vi "main_control_combo_F.vi"(6 "read":bool) -> (9 "chiller actual temperature (C)":string, 10 "bytes read":u32)   [LabVIEW 2019]
doc: "The Basic Serial Read and Write example performs a Serial Port Read, a Serial Port Write, or a combination of these actions. The user selects the actions (read or write) on the front panel. If both are selected, the VI will write the data first, read data, and then close the VISA session that is opened to the port. This VI will wait until the specified number of bytes is received at the port. Only the number of bytes specified will be read.\n\nINSTRUCTIONS:\n1) Select the serial resource and configuration parameters (baud rate, data bits, parity, stop bits, flow control).\n2) Select the operations to be performed. \n3) Connect the serial port to your device. If no device is available, perform a loopback test by doing one of the following. Short pins 2 and 3 on a RS-232 cable or short pin 4 to pin 8 and pin 5 to pin 9 on a RS-485/422 cable. \n4) Run the VI to see the data read. (The \"read string\" will match the \"string to write\" if a loopback test was performed.)\n\nNote: The parameters set for the serial port must match the parameters of the connected instrument or device. In this example, the bytes to read parameter specifies the number of bytes that the serial port reads. If there were more bytes at the port than the number specified in bytes to read, those bytes would not be read. Also, if you specify to read more bytes than the number of bytes actually read, you might receive a timeout error message.\n\nOn the block diagram, the Configure Serial Port VI sets the configuration parameters. The front panel displays the controls used to configure the basic parameters, such as baud rate, data bits, and parity. Constants configure the other parameters the user probably does not need set. After the VISA Configure Serial Port VI opens the VISA session and configures the port, the VI passes the VISA resource name to other VIs that perform operations on that VISA resource. The VISA Write function sends a command to the serial device and the VISA Read function returns data based on the command. The VISA Close function then closes the reference to the serial device. It is important to close the reference; otherwise communication through with that port through protocols other than VISA might not be possible."
uses:
  <vilib>/Instr/_visa.llb/VISA Configure Serial Port (Instr).vi
  <vilib>/Utility/file.llb/Read Delimited Spreadsheet (string).vi
  Keithley/Keithley 24XX/Public/Data/Read (Single Point).vi
  Keithley/Keithley 24XX/Keithley 24XX.lvlib
  <resource>/objmgr/ni.var.rc
panel:
  out "DAQ readout from Linux Box":string
  in  "Output voltage (V)":dbl
  in  "Compliance (A)":dbl=1e-05
  in  "enable manual set":bool
  in  "Reset (default: false)":bool
  out "Finished times":i32
  in  "run single command":bool
  in  "command row":string[](array[string])
  in  "read 4":bool
  in  "read rotronic log manually":bool
  in  "Times to run script":i32=1 caption="times to run script"
  out "COMBO COMMAND":string
  out "manual control":bool
  out "delta actual voltage (V)":string
  in  "delay before read (ms) 4":u32=500
  in  "Combo Box 4":string(combo)
  in  "voltage delta":dbl
  out "delta command":string
  in  "write 4":bool
  in  "stop reading script":bool
  out "dewpoint":string
  out "temperature":string
  out "humidity":string
  out "Voltage (V)":sgl
  out "Current (A)":sgl
  out "Resistance (Om)":sgl
  out "Current (micro amps)":sgl
  out "Command Log and Output":string
  out "all rows":string[][](array[string])
  out "current command":string[](array[string])
  in  "CSV script path":path
  in  "Read Script":bool
  out "relay TTi":errorcluster
  out "bytes read 3":u32
  out "inverter actual voltage":string
  in  "read 3":bool
  in  "delay before read (ms) 3":u32=500
  in  "Combo Box of inverter":string(combo)="VO?\n"
  in  "voltage or current 2":dbl
  out "string from combo 3":string
  in  "write 3":bool
  out "LV TTi":errorcluster
  out "bytes read 2":u32
  out "LVPS actual voltage":string
  in  "read 2":bool
  in  "delay before read (ms) 2":u32=500
  in  "Combo Box of TTi LVPS":string(combo)="VO?\n"
  in  "voltage or current":dbl
  in  "write 2":bool
  in  "write":bool
  out "string from combo":string
  in  "Set Temperature":dbl
  in  "Combo Box of chiller":string(combo)
  out "Chiller":errorcluster
  out "N2 temperature > dew point + 5C":bool
  in  "File Path of rotonic datalog":path
  out "time humidity temporature dewpoint":string[](array[string])
  in  "Quit":bool
  in  "delay before read (ms)":u32=500
  # "Please click \"Reset\" to \"True\" ONLY AFTER Keithley is power cycled\n(BEFORE launching the VI)"
  # "Kiethley Powersupply"
  # "µA"
  # "Delta powersupply Interface"
  # "Medical Chiller\nCOM 6 is default"
  # "TTi LV powersupply\nCOM 5 is default"
  # "TTi LV powersupply for the relay polarity control\nCOM 4 is default"
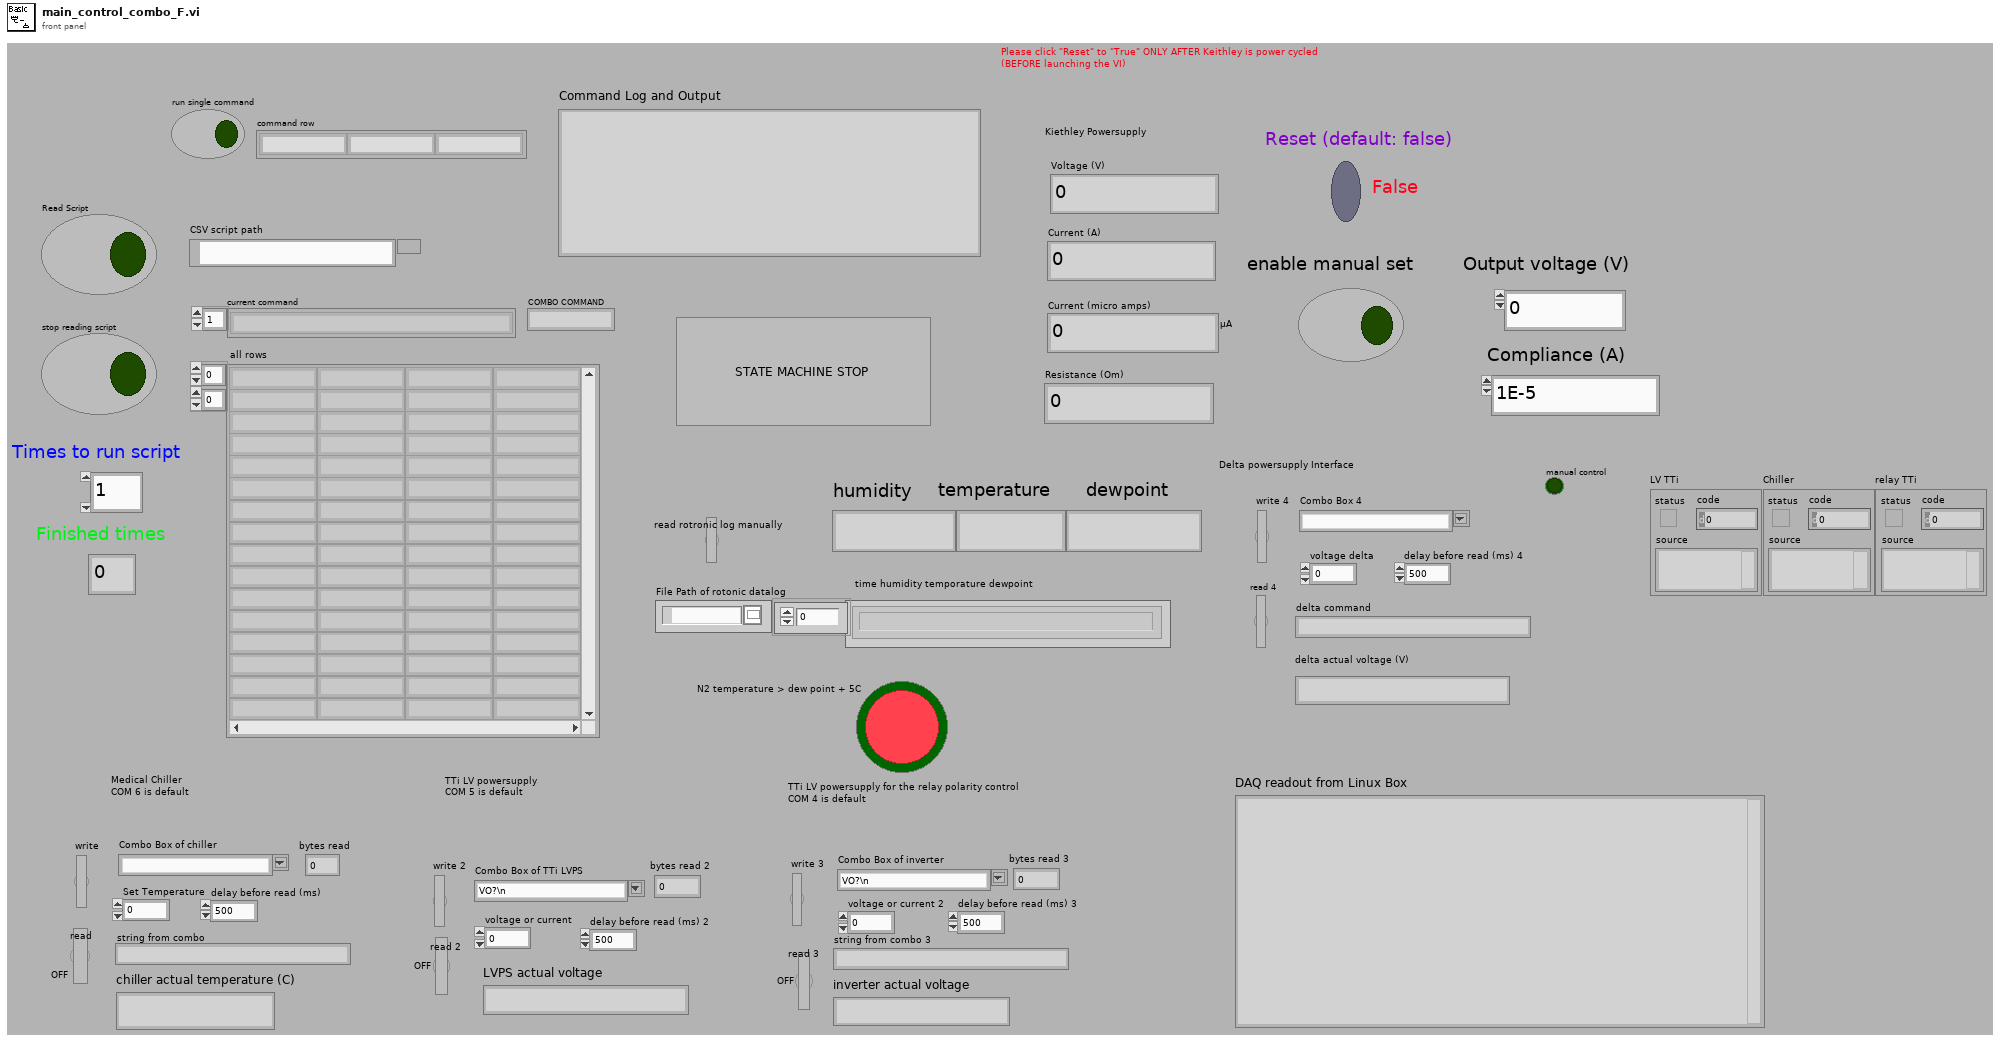
[diagram p1: front panel]
types:
  T1 = cluster{"Baud Rate":u32, "Parity":u16, "Data Bits":u16, "Stop Bits":u16, "Flow Control":u16}
  T2 = enum16{"open", "replace", "create", "open or create", "replace or create", "replace or create with confirmation"}
  T3 = typedef "Semaphore RefNum" = refnum<k1>
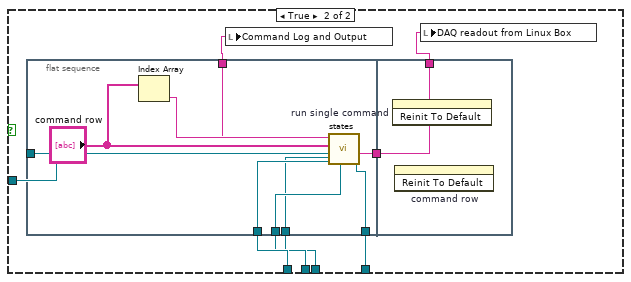
[diagram p3: hidden frame]
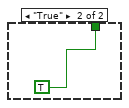
[diagram p4: hidden frame]
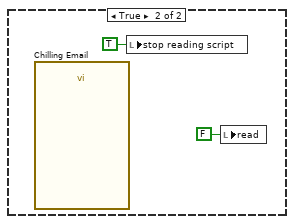
[diagram p6: hidden frame]
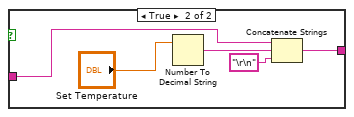
[diagram p7: hidden frame]
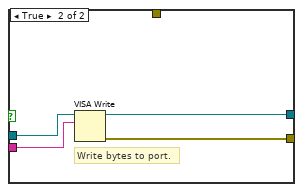
[diagram p8: hidden frame]
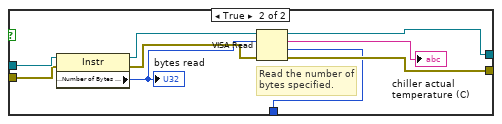
[diagram p9: hidden frame]
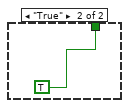
[diagram p10: hidden frame]
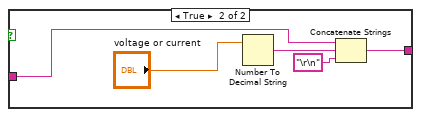
[diagram p12: hidden frame]
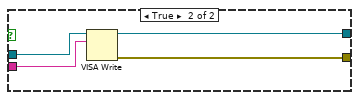
[diagram p13: hidden frame]
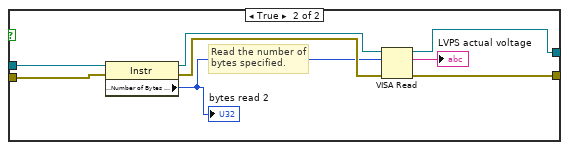
[diagram p14: hidden frame]
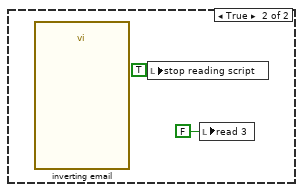
[diagram p16: hidden frame]
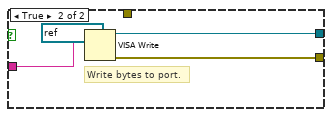
[diagram p18: hidden frame]
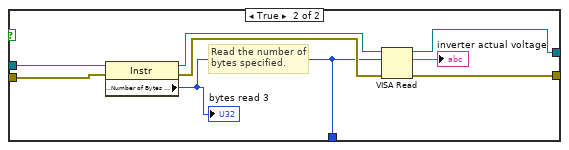
[diagram p19: hidden frame]
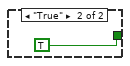
[diagram p20: hidden frame]
diagram:
  # "First save permanent values in non-volatile memory via NI - Max and the *SAV after setting it via SO:VO:MA 52 and SO:CU:MA 30    !"
  n1 = flat-sequence {
    tunnel: [w26] -> w16
    tunnel: [w40] -> w15
    tunnel: [w28] -> w14
    tunnel: [w34] -> w13
    tunnel: [w33] -> w12
    tunnel: [w29] -> w11
    tunnel: [w29] -> w10
    tunnel: [w25] -> w9
    tunnel: [w24] -> w8
    tunnel: [w23] -> w7
    tunnel: [w25] -> w6
    tunnel: [w24] -> w5
    tunnel: [w23] -> w4
    tunnel: [w20] -> w3
    tunnel: [w20] -> w2
    tunnel: [w20] -> w1
    tunnel: [w62] -> w19
    tunnel: [w61] -> w17
    tunnel: w16 -> [w60]
    tunnel: w15 -> [_]
    tunnel: w14 -> [w59]
    tunnel: w13 -> [w57]
    tunnel: w12 -> [w58]
    tunnel: w11 -> [w52]
    tunnel: w10 -> [w56]
    tunnel: w9 -> [w51]
    tunnel: w8 -> [w50]
    tunnel: w7 -> [w49]
    tunnel: w6 -> [w55]
    tunnel: w5 -> [w54]
    tunnel: w4 -> [w53]
    tunnel: w3 -> [w48]
    tunnel: w2 -> [w47]
    tunnel: w1 -> [w46]
    tunnel: w19 -> [w594]
    tunnel: w17 -> [w593]
    frame #0 {
      w27 = refnum<visa-resource-name> "COM4" ("VISA resource name")
      w32 = u32 3000  # timeout (10sec)
      w31 = FALSE  # Enable Termination Char (T)
      w35 = u32 3000  # timeout (10sec)
      w37 = FALSE  # Enable Termination Char (T)
      w38 = u32 3000  # timeout (10sec)
      w41 = FALSE  # Enable Termination Char (T)
      w42 = u32 3000  # timeout (10sec)
      n2 = call "Initialize.vi"("Serial Configuration"=T1 {"Baud Rate"=9600, "Parity"=0, "Data Bits"=8, "Stop Bits"=10, "Flow Control"=1}, "Reset (True)"=FALSE, "VISA resource name"=refnum<visa-resource-name> "COM1" ("VISA resource name 4")) -> ("VISA resource name out"=w21:refnum<visa-resource-name>)  [unwired: 7 in, 1 out]
      n3 = local write "COMBO COMMAND"("" ("COMBO COMMAND")) -> ()
      n4 = VISA Open(timeout (0)=w35, VISA resource name=refnum<visa-resource-name> "GPIB0::8::INSTR") -> (VISA resource name=w34:refnum<visa-resource-name>, error out=w33:errorcluster)  [unwired: 3 in]
      n5 = call-poly "VISA Configure Serial Port"("VISA resource name"=refnum<visa-resource-name> "COM5", "timeout (10sec)"=w38, "Enable Termination\nChar (T)"=w37) -> ("VISA resource name out"=w28:refnum<visa-resource-name>)  [unwired: 11 in, 1 out]
      n6 = call <vilib>:"Obtain Semaphore Reference.vi"("name (unnamed)"=w27) -> ("semaphore"=w24:T3)  [unwired: 4 in, 2 out]
      n7 = call <vilib>:"Obtain Semaphore Reference.vi"("name (unnamed)"=w21) -> ("semaphore"=w20:T3)  [unwired: 4 in, 2 out]
      n8 = call-poly "VISA Configure Serial Port"("VISA resource name"=w27, "timeout (10sec)"=w32, "Enable Termination\nChar (T)"=w31) -> ()  [unwired: 11 in, 2 out]
      n9 = call-poly "VISA Configure Serial Port"("VISA resource name"=refnum<visa-resource-name> "COM6", "timeout (10sec)"=w42, "Enable Termination\nChar (T)"=w41) -> ("VISA resource name out"=w26:refnum<visa-resource-name>, "error out"=w40:errorcluster)  [unwired: 11 in]
      n10 = call <vilib>:"Obtain Semaphore Reference.vi"("name (unnamed)"=w28) -> ("semaphore"=w23:T3)  [unwired: 4 in, 2 out]
      n11 = call <vilib>:"Obtain Semaphore Reference.vi"("name (unnamed)"=w26) -> ("semaphore"=w25:T3)  [unwired: 4 in, 2 out]
      n12 = call <vilib>:"Obtain Semaphore Reference.vi"("name (unnamed)"=w34) -> ("semaphore"=w29:T3)  [unwired: 4 in, 2 out]
    }
    frame #1 {
      # "Disable Output"
      # "State machine for iterating through commands from table"
      n13 = while {
        tunnel: w52 -> [w441]
        tunnel: w51 -> [w440]
        tunnel: w50 -> [w439]
        tunnel: w49 -> [w438]
        tunnel: w47 -> [w437]
        stop <- w443 stop-if-true
        # "keithley"
        # "LV TTi SEH"
        # "inverter"
        # "chiller"
        # "DeltaRef"
        n14 = local read "Quit"() -> (w443:bool)
        n15 = case shown="False" "Read Script" {
          tunnel: "Times to run script" -> [_ w450]
          tunnel: w441 -> [_ w449]
          tunnel: w440 -> [_ w448]
          tunnel: w439 -> [_ w447]
          tunnel: w438 -> [_ w446]
          tunnel: w437 -> [_ w445]
          frame False {
          }
          frame True {
            n16 = Get Date/Time String() -> (date string=w473:string, time string=w471:string)  [unwired: 3 in]
            n17 = Search and Replace String(replace all?=TRUE ("replace all? (F)"), input string=w473, search string="/", replace string="_" ("replace string (\"\")")) -> (result string=w472:string)  [unwired: 4 in, 3 out]
            n18 = Search and Replace String(input string=w471, search string=":", replace string="" ("replace string (\"\")")) -> (result string=w470:string)  [unwired: 5 in, 3 out]
            n19 = Concatenate Strings("C:\\Users\\CMSOTDSF.CERN\\ExecutedCommands\\" ("string"), "command_log_" ("string"), w472, "_" ("string"), w470, ".txt" ("string")) -> (w469:string)
            n20 = String To Path(string=w469) -> (path=w459:path)
            n21 = Open/Create/Replace File(file path (use dialog)=w459, operation (0:open)=T2."replace or create") -> (refnum out=w458:refnum<file>)  [unwired: 4 in, 2 out]
            n22 = Concatenate Strings("Command Log Header for Executed CSV commands " ("text"), "\r\n") -> (w451:string)
            n23 = Set File Position(offset (in bytes) (0)=i64 0, refnum=w458, from (0:start)=enum16{"start", "end", "current"}."end") -> (refnum out=w455:refnum<file>)  [unwired: 1 in, 1 out]
            n24 = Write to Text File(file (use dialog)=w455, text=w451) -> ()  [unwired: 2 in, 3 out]
            n25 = flat-sequence {
              tunnel: w459 -> [w480]
              tunnel: w450 -> [w479]
              tunnel: w449 -> [w478]
              tunnel: w448 -> [w477]
              tunnel: w447 -> [w476]
              tunnel: w446 -> [w475]
              tunnel: w445 -> [w474]
              frame #0 {
                n26 = for {
                  N: w479 -> [_]
                  tunnel: w480 -> [w487]
                  tunnel: w478 -> [w486]
                  tunnel: w477 -> [w485]
                  tunnel: w476 -> [w484]
                  tunnel: w475 -> [w483]
                  tunnel: w474 -> [w481]
                  i -> [w482]
                  n27 = flat-sequence {
                    tunnel: ["CSV script path"] -> w490
                    tunnel: [w493] -> w489
                    tunnel: [w491] -> w488
                    tunnel: w487 -> [w491]
                    tunnel: w490 -> [_]
                    tunnel: w489 -> [w501]
                    tunnel: w488 -> [w500]
                    tunnel: w486 -> [w499]
                    tunnel: w485 -> [w498]
                    tunnel: w484 -> [w497]
                    tunnel: w483 -> [w496]
                    tunnel: w481 -> [w495]
                    frame #0 {
                      # "read table from CSV"
                      n28 = call-poly <vilib>:"Read Delimited Spreadsheet.vi"("file path (dialog if empty)"="CSV script path", "delimiter (\\t)"="," ("delimiter (\\t)")) -> ("all rows"=w493:string[][])  [unwired: 8 in, 5 out]
                    }
                    frame #1 {
                      n29 = Array Size(array=w501) -> (size(s)=w504:i32[])
                      n30 = Index Array(array=w504, index #1=0 ("index"), index #2=1 ("index")) -> (element #1=w505:i32)  [unwired: 1 out]
                      n31 = for {
                        N: w505 -> [_]
                        tunnel: w501 -> [w535] mode=indexing
                        tunnel: w500 -> [w524]
                        tunnel: w499 -> [w514]
                        tunnel: w498 -> [w513]
                        tunnel: w497 -> [w512]
                        tunnel: w496 -> [w511]
                        tunnel: w495 -> [w507]
                        i -> [w522]
                        stop <- w530 stop-if-true
                        n32 = local read "Quit"() -> (w532:bool)
                        n33 = Array Subset(array=w535) -> (w509:string[])  [unwired: 2 in]
                        "current command" <- w509
                        n34 = Or(x=w532, y="stop reading script") -> (x .or. y?=w530:bool)
                        n35 = Array Size(array=w509) -> (size(s)=w534:i32)
                        n36 = Index Array(array=w509, index=0) -> (element=w510:string)
                        "COMBO COMMAND" <- w510
                        n37 = for {
                          N: w534 -> [_]
                          tunnel: w509 -> [w539]
                          tunnel: [w540] -> w515 mode=indexing
                          i -> [w542]
                          n38 = Add(x=w542, y=1) -> (x+y=w538:i32)
                          n39 = Index Array(array=w539, index=w538) -> (element=w537:string)
                          n40 = Wait Until Next ms Multiple(millisecond multiple=u32 1000) -> ()  [unwired: 1 out]
                          n41 = Concatenate Strings(w537, "   " ("string")) -> (w540:string)
                        }
                        n42 = call "states.vi"("keithley"=w507, "LVTTiSEH"=w511, "inverter"=w512, "Chiller"=w513, "DeltaPS"=w514, "Array"=w509, "String"=w510) -> ("From Linux Box"=→"DAQ readout from Linux Box":string, "combo action"=→"Command Log and Output":string)  [unwired: 3 in]
                        n43 = Add(x=w522, y=1) -> (x+y=w520:i32)
                        n44 = Number To Decimal String(number=w520) -> (decimal integer string=w519:string)  [unwired: 1 in]
                        n45 = Open/Create/Replace File(file path (use dialog)=w524, operation (0:open)=T2."open") -> (refnum out=w525:refnum<file>)  [unwired: 4 in, 2 out]
                        n46 = Concatenate Strings(w519, "  " ("string"), w510, "  " ("string"), w515, "\r\n") -> (w523:string)
                        n47 = Set File Position(offset (in bytes) (0)=i64 0, refnum=w525, from (0:start)=enum16{"start", "end", "current"}."end") -> (refnum out=w527:refnum<file>)  [unwired: 1 in, 1 out]
                        n48 = Write to Text File(file (use dialog)=w527, text=w523) -> ()  [unwired: 2 in, 3 out]
                      }
                      "all rows" <- w501
                    }
                  }
                  "Finished times" <- w482
                }
              }
              frame #1 {
                n49 = local write "COMBO COMMAND"("" ("COMBO COMMAND")) -> ()
                n50 = invoke on="Read Script" class="Bool (strict)" method="Reinit To Default"() -> ()  [unwired: 3 in, 3 out]
                n51 = invoke on="stop reading script" class="Bool (strict)" method="Reinit To Default"() -> ()  [unwired: 3 in, 3 out]
              }
            }
          }
        }
      }
      n52 = while {
        tunnel: w57 -> [_]
        tunnel: w58 -> [_]
        tunnel: w56 -> [w308]
        stop <- w322 stop-if-true
        w311 = "True" ("replace string (\"\")")
        n53 = local read "COMBO COMMAND"() -> (w315:string)
        n54 = Search and Replace String(input string=w315, search string="setInverter", replace string=w311) -> (result string=w320:string)  [unwired: 5 in, 3 out]
        n55 = Search and Replace String(input string=w315, search string="setDeltaPS", replace string=w311) -> (result string=w317:string)  [unwired: 5 in, 3 out]
        n56 = case shown="\"False\", Default" w320 {
          tunnel: [FALSE TRUE] -> w321
          frame "False", Default {
          }
          frame "True" {
          }
        }
        n57 = case shown="\"False\", Default" w317 {
          tunnel: [FALSE TRUE] -> w318
          frame "False", Default {
          }
          frame "True" {
          }
        }
        n58 = local read "Quit"() -> (w319:bool)
        n59 = call <vilib>:"Acquire Semaphore.vi"("semaphore"=w308) -> ("error out"=w309:errorcluster, "semaphore out"=w306:T3)  [unwired: 4 in, 1 out]
        n60 = Or(x=w318, y=w319) -> (x .or. y?=w314:bool)
        n61 = Or(x=w314, y=w321) -> (x .or. y?=w313:bool)
        n62 = Not(x=w313) -> (.not. x?=w316:bool)
        "manual control" <- w316
        n63 = case shown="True" w316 {
          tunnel: w309 -> [w325 w331]
          tunnel: [w325 w330] -> w307
          frame False {
          }
          frame True {
            # "delta"
            # "Configure Serial port (baud rate,\ndata bits, parity, stop bits and flow control)."
            n64 = Match True/False String(2:"" ("false string"), 3:"SOUR:VO " ("format string"), 4:"Combo Box 4") -> (0:w336:bool)  [unwired: 1 out]
            n65 = case shown="True" w336 {
              tunnel: [w344 w347] -> w333
              tunnel: "Combo Box 4" -> [w344 w346]
              frame False {
              }
              frame True {
                n66 = Number To Decimal String(number="voltage delta") -> (decimal integer string=w349:string)  [unwired: 1 in]
                n67 = Concatenate Strings(w346, w349, "\n" ("string")) -> (w347:string)
              }
            }
            "delta command" <- w333
            n68 = case shown="True" "write 4" {
              tunnel: [w355 w361] -> w341
              tunnel: [w356 w360] -> w339
              tunnel: w333 -> [_ w359]
              tunnel: w331 -> [w353 _]
              frame False {
                n69 = VISA Write(VISA resource name=refnum<visa-resource-name> "GPIB0::8::INSTR", write buffer="ME:VO?\n", error in (no error)=w353) -> (VISA resource name out=w356:refnum<visa-resource-name>, error out=w355:errorcluster)  [unwired: 1 out]
              }
              frame True {
                # "Write bytes to port."
                n70 = VISA Write(VISA resource name=refnum<visa-resource-name> "GPIB0::8::INSTR", write buffer=w359) -> (VISA resource name out=w360:refnum<visa-resource-name>, error out=w361:errorcluster)  [unwired: 1 in, 1 out]
              }
            }
            n71 = stacked-sequence {
              tunnel: w341 -> [w352]
              tunnel: [w352] -> w340
              tunnel: w339 -> [w351]
              tunnel: [w351] -> w338
              frame #0 {
                n72 = Wait (ms)(milliseconds to wait="delay before read (ms) 4") -> ()  [unwired: 1 out]
              }
            }
            n73 = case shown="False" "read 4" {
              tunnel: w340 -> [w364 w366]
              tunnel: [w364 w371] -> w330
              tunnel: [w363 w370] -> _
              tunnel: w338 -> [w363 w368]
              tunnel: [u32 10 ("return count") w365] -> w328
              frame False {
              }
              frame True {
                # "Read the number of bytes specified."
                n74 = VISA Read(VISA resource name=w368, byte count=u32 1024, error in (no error)=w366) -> (VISA resource name out=w370:refnum<visa-resource-name>, read buffer=→"delta actual voltage (V)":string, return count=w365:u32, error out=w371:errorcluster)
              }
            }
            n75 = Equal?(x=w328, y=0.0) -> (x = y?=w327:bool)
            n76 = case shown="False" w327 {
              frame False {
              }
              frame True {
                n77 = call "delta email"() -> ()  [unwired: 11 in, 1 out]
                n78 = local write "stop reading script"(TRUE ("stop reading script")) -> ()
                n79 = local write "read 4"(FALSE ("read 4")) -> ()
              }
            }
          }
        }
        n80 = local read "Quit"() -> (w322:bool)
        n81 = call <vilib>:"Release Semaphore.vi"("error in (no error)"=w307, "semaphore"=w306) -> ()  [unwired: 4 in, 2 out]
      }
      n82 = while {
        stop <- "Quit" stop-if-true
      }
      n83 = while {
        tunnel: w59 -> [w194]
        tunnel: [w195] -> w62
        tunnel: w53 -> [w183]
        stop <- w193 stop-if-true
        n84 = local read "COMBO COMMAND"() -> (w185:string)
        n85 = call <vilib>:"Acquire Semaphore.vi"("semaphore"=w183) -> ("error out"=w182:errorcluster, "semaphore out"=w180:T3)  [unwired: 4 in, 1 out]
        n86 = Search and Replace String(input string=w185, search string="setLVPS", replace string="True" ("replace string (\"\")")) -> (result string=w190:string)  [unwired: 5 in, 3 out]
        n87 = case shown="\"False\", Default" w190 {
          tunnel: [FALSE TRUE] -> w191
          frame "False", Default {
          }
          frame "True" {
          }
        }
        n88 = local read "Quit"() -> (w192:bool)
        n89 = Or(x=w191, y=w192) -> (x .or. y?=w187:bool)
        n90 = Not(x=w187) -> (.not. x?=w186:bool)
        n91 = case shown="True" w186 {
          tunnel: [w198 w214] -> w181
          tunnel: [w199 w213] -> w195
          tunnel: w194 -> [w199 w212]
          tunnel: w182 -> [w198 w200]
          frame False {
          }
          frame True {
            # "TTi SEH PS LV"
            n92 = Match True/False String(2:"" ("false string"), 3:"OUT_SP_00_" ("format string"), 4:"Combo Box of TTi LVPS") -> (0:w205:bool)  [unwired: 1 out]
            n93 = case shown="False" w205 {
              tunnel: [w215 w218] -> w202
              tunnel: "Combo Box of TTi LVPS" -> [w215 w217]
              frame False {
              }
              frame True {
                n94 = Number To Decimal String(number="voltage or current") -> (decimal integer string=w220:string)  [unwired: 1 in]
                n95 = Concatenate Strings(w217, w220, "\r\n" ("string")) -> (w218:string)
              }
            }
            n96 = case shown="False" "write 2" {
              tunnel: [w225 w232] -> w210
              tunnel: w212 -> [w227 w231]
              tunnel: [w226 w230] -> w208
              tunnel: w202 -> [_ w229]
              tunnel: w200 -> [w224 _]
              frame False {
                n97 = VISA Write(VISA resource name=w227, write buffer="VO?\n", error in (no error)=w224) -> (VISA resource name out=w226:refnum<visa-resource-name>, error out=w225:errorcluster)  [unwired: 1 out]
              }
              frame True {
                n98 = VISA Write(VISA resource name=w231, write buffer=w229) -> (VISA resource name out=w230:refnum<visa-resource-name>, error out=w232:errorcluster)  [unwired: 1 in, 1 out]
              }
            }
            n99 = stacked-sequence {
              tunnel: w210 -> [w223]
              tunnel: [w223] -> w209
              tunnel: w208 -> [w222]
              tunnel: [w222] -> w207
              frame #0 {
                n100 = Wait (ms)(milliseconds to wait="delay before read (ms) 2") -> ()  [unwired: 1 out]
              }
            }
            n101 = case shown="False" "read 2" {
              tunnel: w209 -> [w234 w238]
              tunnel: [w234 w242] -> w214
              tunnel: [w233 w241] -> w213
              tunnel: w207 -> [w233 w240]
              frame False {
              }
              frame True {
                # "Read the number of bytes specified."
                n102 = property class="Instr"(reference=w240, error in=w238) -> (reference out=w239:refnum<visa-resource-name>, error out=w237:errorcluster, "Serial Settings:Number of Bytes at Serial Port"=w236:u32)
                "bytes read 2" <- w236
                n103 = VISA Read(VISA resource name=w239, byte count=w236, error in (no error)=w237) -> (VISA resource name out=w241:refnum<visa-resource-name>, read buffer=→"LVPS actual voltage":string, error out=w242:errorcluster)  [unwired: 1 out]
              }
            }
          }
        }
        n104 = call <vilib>:"Release Semaphore.vi"("error in (no error)"=w181, "semaphore"=w180) -> ()  [unwired: 4 in, 2 out]
        n105 = local read "Quit"() -> (w193:bool)
        n106 = Wait Until Next ms Multiple(millisecond multiple=u32 1000) -> ()  [unwired: 1 out]
      }
      n107 = while {
        tunnel: w54 -> [w246]
        stop <- w255 stop-if-true
        # "TTi Inverter for Relay"
        n108 = local read "COMBO COMMAND"() -> (w253:string)
        n109 = call <vilib>:"Acquire Semaphore.vi"("semaphore"=w246) -> ("error out"=w243:errorcluster, "semaphore out"=w245:T3)  [unwired: 4 in, 1 out]
        n110 = Search and Replace String(input string=w253, search string="setInverter", replace string="True" ("replace string (\"\")")) -> (result string=w249:string)  [unwired: 5 in, 3 out]
        n111 = case shown="\"False\", Default" w249 {
          tunnel: [FALSE TRUE] -> w250
          frame "False", Default {
          }
          frame "True" {
          }
        }
        n112 = local read "Quit"() -> (w251:bool)
        n113 = Or(x=w250, y=w251) -> (x .or. y?=w252:bool)
        n114 = Not(x=w252) -> (.not. x?=w254:bool)
        n115 = case shown="True" w254 {
          tunnel: [w256 w261] -> w244
          tunnel: w243 -> [w256 w260]
          frame False {
          }
          frame True {
            # "Configure Serial port (baud rate,\ndata bits, parity, stop bits and flow control)."
            n116 = Match True/False String(2:"" ("false string"), 3:"OUT_SP_00_" ("format string"), 4:"Combo Box of inverter") -> (0:w270:bool)  [unwired: 1 out]
            n117 = case shown="True" w270 {
              tunnel: [w275 w278] -> w271
              tunnel: "Combo Box of inverter" -> [w275 w277]
              frame False {
              }
              frame True {
                n118 = Number To Decimal String(number="voltage or current 2") -> (decimal integer string=w280:string)  [unwired: 1 in]
                n119 = Concatenate Strings(w277, w280, "\r\n" ("string")) -> (w278:string)
              }
            }
            "string from combo 3" <- w271
            n120 = case shown="False" "write 3" {
              tunnel: [w286 w292] -> w265
              tunnel: [w287 w291] -> w267
              tunnel: w271 -> [_ w290]
              tunnel: w260 -> [w284 _]
              frame False {
                n121 = VISA Write(VISA resource name=refnum<visa-resource-name> "COM4", write buffer="VO?\n", error in (no error)=w284) -> (VISA resource name out=w287:refnum<visa-resource-name>, error out=w286:errorcluster)  [unwired: 1 out]
              }
              frame True {
                # "Write bytes to port."
                n122 = VISA Write(VISA resource name=refnum<visa-resource-name> "COM4", write buffer=w290) -> (VISA resource name out=w291:refnum<visa-resource-name>, error out=w292:errorcluster)  [unwired: 1 in, 1 out]
              }
            }
            n123 = stacked-sequence {
              tunnel: w265 -> [w283]
              tunnel: [w283] -> w266
              tunnel: w267 -> [w282]
              tunnel: [w282] -> w268
              frame #0 {
                n124 = Wait (ms)(milliseconds to wait="delay before read (ms) 3") -> ()  [unwired: 1 out]
              }
            }
            n125 = case shown="False" "read 3" {
              tunnel: w266 -> [w295 w299]
              tunnel: [w295 w303] -> w261
              tunnel: [w294 w302] -> _
              tunnel: w268 -> [w294 w301]
              tunnel: [u32 10 ("Bytes at Port") w296] -> w258
              frame False {
              }
              frame True {
                # "Read the number of bytes specified."
                n126 = property class="Instr"(reference=w301, error in=w299) -> (reference out=w300:refnum<visa-resource-name>, error out=w298:errorcluster, "Serial Settings:Number of Bytes at Serial Port"=w296:u32)
                "bytes read 3" <- w296
                n127 = VISA Read(VISA resource name=w300, byte count=w296, error in (no error)=w298) -> (VISA resource name out=w302:refnum<visa-resource-name>, read buffer=→"inverter actual voltage":string, error out=w303:errorcluster)  [unwired: 1 out]
              }
            }
            n128 = Equal?(x=w258, y=0.0) -> (x = y?=w257:bool)
            n129 = case shown="False" w257 {
              frame False {
              }
              frame True {
                n130 = call "inverting email"() -> ()  [unwired: 11 in, 1 out]
                n131 = local write "stop reading script"(TRUE ("stop reading script")) -> ()
                n132 = local write "read 3"(FALSE ("read 3")) -> ()
              }
            }
          }
        }
        n133 = call <vilib>:"Release Semaphore.vi"("error in (no error)"=w244, "semaphore"=w245) -> ()  [unwired: 4 in, 2 out]
        n134 = local read "Quit"() -> (w255:bool)
      }
      n135 = while {
        tunnel: w60 -> [w124]
        tunnel: [w125] -> w61
        tunnel: w55 -> [w113]
        stop <- w123 stop-if-true
        n136 = local read "COMBO COMMAND"() -> (w115:string)
        n137 = call <vilib>:"Acquire Semaphore.vi"("semaphore"=w113) -> ("error out"=w112:errorcluster, "semaphore out"=w111:T3)  [unwired: 4 in, 1 out]
        n138 = Search and Replace String(input string=w115, search string="setChiller", replace string="True" ("replace string (\"\")")) -> (result string=w120:string)  [unwired: 5 in, 3 out]
        n139 = case shown="\"False\", Default" w120 {
          tunnel: [FALSE TRUE] -> w121
          frame "False", Default {
          }
          frame "True" {
          }
        }
        n140 = local read "Quit"() -> (w122:bool)
        n141 = Or(x=w121, y=w122) -> (x .or. y?=w117:bool)
        n142 = Not(x=w117) -> (.not. x?=w116:bool)
        n143 = case shown="True" w116 {
          tunnel: [w129 w147] -> w125
          tunnel: w124 -> [w129 w146]
          tunnel: w112 -> [w128 w131]
          tunnel: [w128 w130] -> w110
          frame False {
          }
          frame True {
            # "CHILLER"
            # "Configure Serial port (baud rate,\ndata bits, parity, stop bits and flow control)."
            n144 = Match True/False String(2:"" ("false string"), 3:"OUT_SP_00_" ("format string"), 4:"Combo Box of chiller") -> (0:w139:bool)  [unwired: 1 out]
            n145 = case shown="False" w139 {
              tunnel: [w150 w153] -> w136
              tunnel: "Combo Box of chiller" -> [w150 w152]
              frame False {
              }
              frame True {
                n146 = Number To Decimal String(number="Set Temperature") -> (decimal integer string=w155:string)  [unwired: 1 in]
                n147 = Concatenate Strings(w152, w155, "\r\n" ("string")) -> (w153:string)
              }
            }
            "string from combo" <- w136
            n148 = case shown="False" "write" {
              tunnel: [w160 w167] -> w144
              tunnel: w146 -> [w163 w166]
              tunnel: [w161 w165] -> w142
              tunnel: w136 -> [_ w164]
              tunnel: w131 -> [w159 _]
              frame False {
                n149 = VISA Write(VISA resource name=w163, write buffer="IN_PV_00\r\n", error in (no error)=w159) -> (VISA resource name out=w161:refnum<visa-resource-name>, error out=w160:errorcluster)  [unwired: 1 out]
              }
              frame True {
                # "Write bytes to port."
                n150 = VISA Write(VISA resource name=w166, write buffer=w164) -> (VISA resource name out=w165:refnum<visa-resource-name>, error out=w167:errorcluster)  [unwired: 1 in, 1 out]
              }
            }
            n151 = stacked-sequence {
              tunnel: w144 -> [w158]
              tunnel: [w158] -> w143
              tunnel: w142 -> [w157]
              tunnel: [w157] -> w141
              frame #0 {
                n152 = Wait (ms)(milliseconds to wait="delay before read (ms)") -> ()  [unwired: 1 out]
              }
            }
            n153 = case shown="False" "read" {
              tunnel: w143 -> [w170 w175]
              tunnel: [w170 w179] -> w130
              tunnel: [w169 w178] -> w147
              tunnel: w141 -> [w169 w177]
              tunnel: [u32 10 ("return count") w171] -> w133
              frame False {
              }
              frame True {
                # "Read the number of bytes specified."
                n154 = property class="Instr"(reference=w177, error in=w175) -> (reference out=w176:refnum<visa-resource-name>, error out=w174:errorcluster, "Serial Settings:Number of Bytes at Serial Port"=w173:u32)
                "bytes read" <- w173
                n155 = VISA Read(VISA resource name=w176, byte count=w173, error in (no error)=w174) -> (VISA resource name out=w178:refnum<visa-resource-name>, read buffer=→"chiller actual temperature (C)":string, return count=w171:u32, error out=w179:errorcluster)
              }
            }
            n156 = Equal?(x=w133, y=0.0) -> (x = y?=w132:bool)
            n157 = case shown="False" w132 {
              frame False {
              }
              frame True {
                n158 = call "Chilling Email"() -> ()  [unwired: 11 in, 1 out]
                n159 = local write "stop reading script"(TRUE ("stop reading script")) -> ()
                n160 = local write "read"(FALSE ("read")) -> ()
              }
            }
          }
        }
        n161 = local read "Quit"() -> (w123:bool)
        n162 = Wait Until Next ms Multiple(millisecond multiple=u32 1000) -> ()  [unwired: 1 out]
        n163 = call <vilib>:"Release Semaphore.vi"("error in (no error)"=w110, "semaphore"=w111) -> ()  [unwired: 4 in, 2 out]
      }
      n164 = while {
        stop <- w547 stop-if-true
        # "dew point"
        # "N2 flow temperature"
        # "Convert text file string to array"
        # "Return the Number of lines."
        # "Extract only the size dimension we need"
        # "Get the size of the array"
        # "Read Text File, dialog box if none"
        n165 = case shown="False" "read rotronic log manually" {
          tunnel: [w586 "File Path of rotonic datalog"] -> w545
          frame False {
            n166 = Get Date/Time In Seconds() -> (seconds since 1Jan1904=w585:timestamp)
            n167 = Format Date/Time String(time format string (%c)="%Y%m%d.xls", seconds (now)=w585) -> (date/time string=w583:string)  [unwired: 1 in]
            n168 = Concatenate Strings("C:\\Users\\CMSOTDSF.CERN\\Desktop\\rotronic_readout\\humidity_" ("time format string (%c)"), w583) -> (w587:string)
            n169 = String To Path(string=w587) -> (path=w586:path)
          }
          frame True {
          }
        }
        n170 = local read "Quit"() -> (w547:bool)
        n171 = Read from Text File(file (use dialog)=w545) -> (text=w574:string)  [unwired: 1 in, 5 out]
        n172 = Spreadsheet String To Array(delimiter (Tab)="\r", format string="%d", spreadsheet string=w574) -> (array=w572:dbl[][])  [unwired: 1 out]
        n173 = Array Size(array=w572) -> (size(s)=w573:i32[])
        n174 = Index Array(array=w573) -> (element=w576:i32)  [unwired: 1 in]
        n175 = Read from Text File(file (use dialog)=w545, count=w576) -> (text=w577:string[])  [unwired: 1 in, 4 out]
        n176 = Decrement(x=w576) -> (x-1=w575:i32)
        n177 = Array Subset(array=w577, index=w575) -> (w578:string[])  [unwired: 1 in]
        "time humidity temporature dewpoint" <- w578
        n178 = Get Date/Time In Seconds() -> (seconds since 1Jan1904=w570:timestamp)
        n179 = Array To Spreadsheet String(array=w578, 3:"%d/%m/%Y %H:%M:%S %4.12f %4.12f %4.12f" ("time format string (%c)")) -> (spreadsheet string=w549:string)  [unwired: 1 in]
        n180 = Format Date/Time String(time format string (%c)="%d/%m/%Y %H:%M:%S ", seconds (now)=w570) -> (date/time string=w571:string)  [unwired: 1 in]
        n181 = String Subset(string=w549, offset (0)=20, length (rest)=5 ("length (rest)")) -> (substring=→"humidity":string)
        n182 = Scan From String(format string=w571, input string=w549) -> (remaining string=w579:string)  [unwired: 4 in, 2 out]
        n183 = String Subset(string=w549, offset (0)=27, length (rest)=5 ("length (rest)")) -> (substring=→"temperature":string)
        n184 = String Subset(string=w549, offset (0)=34, length (rest)=6 ("length (rest)")) -> (substring=w548:string)
        "dewpoint" <- w548
        n185 = property class="Variable Object" props=["ClassId"](reference=w548) -> ()  [unwired: 1 in, 3 out]
        n186 = String Subset(string=w579, offset (0)=12, length (rest)=5 ("length (rest)")) -> (substring=w580:string)
        n187 = Fract/Exp String To Number(string=w580) -> (number=w560:dbl)  [unwired: 3 in, 1 out]
        n188 = String Subset(string=w579, offset (0)=6, length (rest)=5 ("length (rest)")) -> (substring=w558:string)
        n189 = Fract/Exp String To Number(string=w558) -> (number=w581:dbl)  [unwired: 3 in, 1 out]
        n190 = Add(x=w560, y=5.0) -> (x+y=w559:dbl)
        n191 = Greater?(x=w581, y=w559) -> (0:→"N2 temperature > dew point + 5C":bool)
        n192 = call <vilib>:"Simple Error Handler.vi"() -> ()  [unwired: 5 in, 5 out]
      }
      n193 = while {
        stop <- w375 stop-if-true
        n194 = local read "CSV script path"() -> (w376:path)
        n195 = Equal?(x=w376, y=path "") -> (x = y?=w380:bool)
        n196 = case shown="False" w380 {
          tunnel: [w382 path "C:/LabVIEW/OuterTrackerControl/example_commands.csv"] -> w381
          tunnel: w376 -> [w382 _]
          frame False {
          }
          frame True {
          }
        }
        n197 = local read "Quit"() -> (w375:bool)
        n198 = call-poly <vilib>:"Read Delimited Spreadsheet.vi"("file path (dialog if empty)"=w381, "delimiter (\\t)"="," ("delimiter (\\t)")) -> ("all rows"=w379:string[][])  [unwired: 8 in, 5 out]
        n199 = local write "all rows"(w379) -> ()
      }
      n200 = while {
        tunnel: w48 -> [w392]
        stop <- w389 stop-if-true
        # "Take the readings."
        # "Configure the output."
        # "Configure each of the three measurements. settings"
        n201 = call <vilib>:"Acquire Semaphore.vi"("semaphore"=w392) -> ("error out"=w391:errorcluster, "semaphore out"=w384:T3)  [unwired: 4 in, 1 out]
        n202 = local read "COMBO COMMAND"() -> (w393:string)
        n203 = Search and Replace String(input string=w393, search string="keithleynew", replace string="True" ("replace string (\"\")")) -> (result string=w395:string)  [unwired: 5 in, 3 out]
        n204 = case shown="\"False\", Default" w395 {
          tunnel: [FALSE TRUE] -> w394
          frame "False", Default {
          }
          frame "True" {
          }
        }
        n205 = local read "Quit"() -> (w386:bool)
        n206 = Or(x=w386, y=w394) -> (x .or. y?=w388:bool)
        n207 = Not(x=w388) -> (.not. x?=w387:bool)
        n208 = case shown="True" w387 {
          tunnel: w391 -> [w398 w416]
          tunnel: [w398 w415] -> w390
          frame False {
          }
          frame True {
            w410 = u16 2 items=["Volts", "Current", "Resistance"] ("Function (0: Volts)")
            w413 = u16 1 items=["Volts", "Current", "Resistance"] ("Function (0: Volts)")
            w426 = u16 0 items=["Volts", "Current", "Resistance"]  # Function (0: Volts)
            n209 = call "Configure Measurement.vi"("Manual Range (1.0)"=1.0, "error in (no error)"=w416, "Function (0: Volts)"=w426, "VISA resource name"=refnum<visa-resource-name> "COM1") -> ("error out"=w412:errorcluster, "VISA resource name out"=w414:refnum<visa-resource-name>)  [unwired: 6 in]
            n210 = call "Configure Measurement.vi"("Manual Range (1.0)"=1e-05, "error in (no error)"=w412, "Function (0: Volts)"=w413, "VISA resource name"=w414) -> ("error out"=w409:errorcluster, "VISA resource name out"=w411:refnum<visa-resource-name>)  [unwired: 6 in]
            n211 = call "Configure Measurement.vi"("Manual Range (1.0)"=1.0, "error in (no error)"=w409, "Function (0: Volts)"=w410, "VISA resource name"=w411) -> ("error out"=w403:errorcluster, "VISA resource name out"=w404:refnum<visa-resource-name>)  [unwired: 6 in]
            n212 = case shown="True" "enable manual set" {
              tunnel: w404 -> [w428 w434]
              tunnel: w403 -> [w427 w433]
              tunnel: [w428 w432] -> w402
              tunnel: [w427 w431] -> w401
              tunnel: "Compliance (A)" -> [_ w430]
              tunnel: "Output voltage (V)" -> [_ w429]
              frame False {
              }
              frame True {
                n213 = call "Configure Output.vi"("error in (no error)"=w433, "Compliance  Level (0.1)"=w430, "Output Level (0)"=w429, "VISA resource name"=w434) -> ("error out"=w431:errorcluster, "VISA resource name out"=w432:refnum<visa-resource-name>)  [unwired: 6 in]
              }
            }
            n214 = call "Enable Output.vi"("error in (no error)"=w401, "Enable Output (T: Enable)"=TRUE, "VISA resource name"=w402) -> ("error out"=w419:errorcluster, "VISA resource name out"=w418:refnum<visa-resource-name>)  [unwired: 7 in]
            n215 = call-poly "Read.vi"("VISA resource name"=w418, "error in (no error)"=w419) -> ("Voltage"=→"Voltage (V)":sgl, "Current"=w424:sgl, "Resistance"=→"Resistance (Om)":sgl, "error out"=w415:errorcluster)  [unwired: 7 in, 3 out]
            "Current (A)" <- w424
            n216 = Multiply(x=w424, y=sgl 1000000.0) -> (x*y=→"Current (micro amps)":sgl)
          }
        }
        n217 = call <vilib>:"Release Semaphore.vi"("error in (no error)"=w390, "semaphore"=w384) -> ()  [unwired: 4 in, 2 out]
        n218 = Wait Until Next ms Multiple(millisecond multiple=u32 1000) -> ()  [unwired: 1 out]
        n219 = local read "Quit"() -> (w389:bool)
      }
      n220 = while {
        tunnel: w52 -> [w91]
        tunnel: w51 -> [w90]
        tunnel: w50 -> [w89]
        tunnel: w49 -> [w88]
        tunnel: w47 -> [w85]
        stop <- w87 stop-if-true
        n221 = case shown="False" "run single command" {
          tunnel: w91 -> [_ w99]
          tunnel: w90 -> [_ w98]
          tunnel: w89 -> [_ w97]
          tunnel: w88 -> [_ w96]
          tunnel: w85 -> [_ w95]
          frame False {
          }
          frame True {
            n222 = flat-sequence {
              tunnel: w99 -> [w108]
              tunnel: w98 -> [w107]
              tunnel: w97 -> [w106]
              tunnel: w96 -> [w105]
              tunnel: w95 -> [w102]
              tunnel: [w101] -> w94
              tunnel: [w100] -> w93
              tunnel: [w109] -> w92
              tunnel: w94 -> [w109]
              frame #0 {
                n223 = Index Array(array="command row") -> (element=w104:string)  [unwired: 1 in]
                n224 = call "states.vi"("keithley"=w102, "LVTTiSEH"=w105, "inverter"=w106, "Chiller"=w107, "DeltaPS"=w108, "Array"="command row", "String"=w104) -> ("From Linux Box"=w101:string, "combo action"=w100:string)  [unwired: 3 in]
              }
              frame #1 {
                n225 = invoke on="run single command" class="Bool (strict)" method="Reinit To Default"() -> ()  [unwired: 3 in, 3 out]
                n226 = invoke on="command row" class="Arr (strict)" method="Reinit To Default"() -> ()  [unwired: 3 in, 3 out]
              }
            }
            n227 = local write "Command Log and Output"(w93) -> ()
            n228 = local write "DAQ readout from Linux Box"(w92) -> ()
          }
        }
        n229 = local read "Quit"() -> (w87:bool)
      }
      n230 = while {
        tunnel: w46 -> [w64]
        stop <- w67 stop-if-true
        n231 = call <vilib>:"Acquire Semaphore.vi"("semaphore"=w64) -> ("error out"=w66:errorcluster, "semaphore out"=w63:T3)  [unwired: 4 in, 1 out]
        n232 = case shown="True" "Reset (default: false)" {
          tunnel: w66 -> [w69 w71]
          tunnel: [w69 w70] -> w65
          frame False {
          }
          frame True {
            n233 = flat-sequence {
              tunnel: w71 -> [w73]
              tunnel: [w72] -> w70
              frame #0 {
                w76 = u16 0 items=["Voltage", "Current"] ("Source Mode  (0: Voltage)")
                n234 = call "Initialize.vi"("Serial Configuration"=T1 {"Baud Rate"=9600, "Parity"=0, "Data Bits"=8, "Stop Bits"=10, "Flow Control"=1}, "error in (no error)"=w73, "Reset (True)"=TRUE, "VISA resource name"=refnum<visa-resource-name> "COM1" ("VISA resource name 4")) -> ("error out"=w79:errorcluster, "VISA resource name out"=w80:refnum<visa-resource-name>)  [unwired: 6 in]
                n235 = call "Configure Output.vi"("Source Mode  (0: Voltage)"=w76, "error in (no error)"=w79, "Compliance  Level (0.1)"=1e-05, "VISA resource name"=w80) -> ("error out"=w77:errorcluster, "VISA resource name out"=w78:refnum<visa-resource-name>)  [unwired: 6 in]
                n236 = call "Enable Output.vi"("error in (no error)"=w77, "Enable Output (T: Enable)"=FALSE, "VISA resource name"=w78) -> ("error out"=w72:errorcluster)  [unwired: 7 in, 1 out]
              }
              frame #1 {
                n237 = local write "Reset (default: false)"(FALSE ("Reset (default: false)")) -> ()
              }
            }
          }
        }
        n238 = local read "Quit"() -> (w67:bool)
        n239 = call <vilib>:"Release Semaphore.vi"("error in (no error)"=w65, "semaphore"=w63) -> ()  [unwired: 4 in, 2 out]
      }
    }
    frame #2 {
      # "Closing things down"
      n240 = VISA Close(VISA resource name=w594) -> (error out=w595:errorcluster)  [unwired: 1 in]
      "LV TTi" <- w595
      n241 = VISA Close(VISA resource name=refnum<visa-resource-name> "GPIB0::8::INSTR") -> ()  [unwired: 1 in, 1 out]
      n242 = call <vilib>:"Simple Error Handler.vi"("error in (no error)"=w595) -> ()  [unwired: 4 in, 5 out]
      n243 = call "Close.vi"("VISA resource name"=refnum<visa-resource-name> "COM1" ("VISA resource name 4")) -> ()  [unwired: 10 in, 1 out]
      n244 = VISA Close(VISA resource name=refnum<visa-resource-name> "COM4") -> (error out=w596:errorcluster)  [unwired: 1 in]
      "relay TTi" <- w596
      n245 = VISA Close(VISA resource name=w593) -> (error out=w597:errorcluster)  [unwired: 1 in]
      "Chiller" <- w597
      n246 = call <vilib>:"Simple Error Handler.vi"("error in (no error)"=w596) -> ()  [unwired: 4 in, 5 out]
      n247 = call <vilib>:"Simple Error Handler.vi"("error in (no error)"=w597) -> ()  [unwired: 4 in, 5 out]
    }
  }
  n248 = property on="dewpoint" class="Str"("Text.FontSize"=u32 30 ("Text.Font:Size")) -> ()  [unwired: 2 in, 2 out]
